vi "Translator.ControlTypeCheck.vi"(1 "control ref":refnum<vi>) -> (0 "control type":T1)   [LabVIEW 2019, in "Tools.lvlib"]
uses:
  Tools.lvlib
  Translator.ControlTypes.ctl
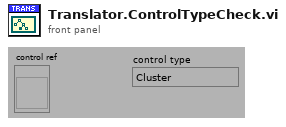
[diagram p1: front panel]
types:
  T1 = typedef "Tools.lvlib/Translator.ControlTypes.ctl" = enum16{"Cluster", "Array", "Boolean", "Ring", "String", "Tab", "Listbox", "Multicolumn listbox", "Table", "Other"}
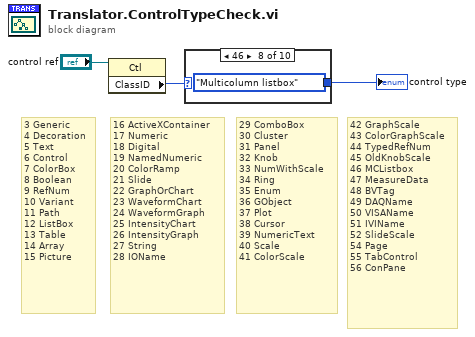
[diagram p0: block diagram]
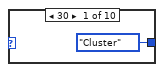
[diagram p2: hidden frame]
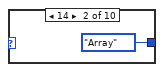
[diagram p3: hidden frame]
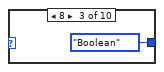
[diagram p4: hidden frame]
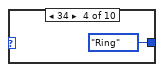
[diagram p5: hidden frame]
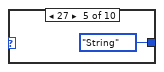
[diagram p6: hidden frame]
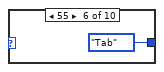
[diagram p7: hidden frame]
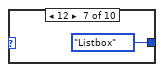
[diagram p8: hidden frame]
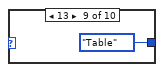
[diagram p9: hidden frame]
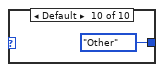
[diagram p10: hidden frame]
diagram:
  # "42 GraphScale \n43 ColorGraphScale \n44 TypedRefNum \n45 OldKnobScale \n46 MCListbox \n47 MeasureData \n48 BVTag \n49 DAQName \n50 VISAName \n51 IVIName \n52 SlideScale \n54 Page \n55 TabControl \n56 ConPane"
  # "16 ActiveXContainer \n17 Numeric \n18 Digital \n19 NamedNumeric \n20 ColorRamp \n21 Slide \n22 GraphOrChart \n23 WaveformChart \n24 WaveformGraph \n25 IntensityChart \n26 IntensityGraph \n27 String \n28 IOName"
  # "29 ComboBox \n30 Cluster \n31 Panel \n32 Knob \n33 NumWithScale \n34 Ring \n35 Enum \n36 GObject \n37 Plot \n38 Cursor \n39 NumericText \n40 Scale \n41 ColorScale"
  # "3 Generic \n4 Decoration \n5 Text \n6 Control \n7 ColorBox \n8 Boolean \n9 RefNum \n10 Variant \n11 Path \n12 ListBox \n13 Table \n14 Array \n15 Picture"
  n1 = property class="Ctl"(reference="control ref") -> ("ClassID"=w2:u32)  [unwired: 1 in, 2 out]
  n2 = case shown="46" w2 {
    tunnel: [Translator.ControlTypes."Cluster" ("control type") Translator.ControlTypes."Array" ("control type") Translator.ControlTypes."Boolean" ("control type") Translator.ControlTypes."Ring" ("control type") Translator.ControlTypes."String" ("control type") Translator.ControlTypes."Tab" ("control type") Translator.ControlTypes."Listbox" ("control type") Translator.ControlTypes."Multicolumn listbox" ("control type") Translator.ControlTypes."Table" ("control type") Translator.ControlTypes."Other" ("control type")] -> w1
    frame 30 {
    }
    frame 14 {
    }
    frame 8 {
    }
    frame 34 {
    }
    frame 27 {
    }
    frame 55 {
    }
    frame 12 {
    }
    frame 46 {
    }
    frame 13 {
    }
    frame Default {
    }
  }
  "control type" <- w1
